vi "Init.vi"(7 "Obj Dict":refnum<class "Object Dictionary.lvclass">, 8 "error in":errorcluster, 10 "OD Entry":refnum<class "Object Entry.lvclass">, 11 "RPDO Mapping in":refnum<class "RPDO Mapping.lvclass">) -> (0 "error out":errorcluster, 3 "RPDO Mapping out":refnum<class "RPDO Mapping.lvclass">)   [LabVIEW 2020, in "CANopen.lvlib" / "RPDO Mapping.lvclass"]
uses:
  RPDO Mapping.lvclass
  Object Entry/Object Entry.lvclass
  Object Dictionary/Object Dictionary.lvclass
  PDO Mapping/PDO Mapping.lvclass
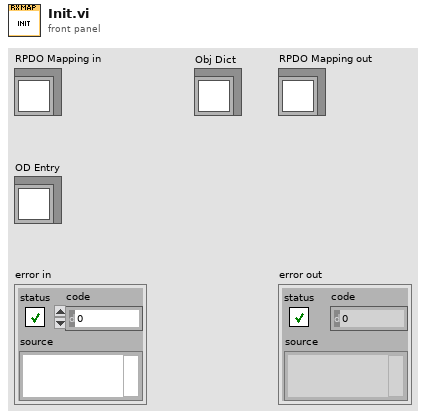
[diagram p1: front panel]
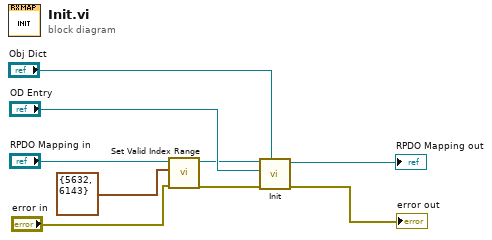
[diagram p0: block diagram]
diagram:
  n1 = call "Set Valid Index Range.vi"("error in"="error in", "Valid Index Range"=cluster{"Lower":u16, "Upper":u16} {"Lower"=5632, "Upper"=6143}, "PDO Mapping in"="RPDO Mapping in") -> ("error out"=w4:errorcluster, "PDO Mapping out"=w2:refnum<class "RPDO Mapping.lvclass">)  [unwired: 7 in]
  n2 = call-parent "Init.vi"("Obj Dict"="Obj Dict", "error in"=w4, "OD Entry"="OD Entry", "PDO Mapping in"=w2) -> ("error out"=→"error out":errorcluster, "PDO Mapping out"=→"RPDO Mapping out":refnum<class "RPDO Mapping.lvclass">)  [unwired: 6 in]
